vi "Action Name.vi"(11 "InitAction in":refnum<class "InitAction.lvclass">) -> (2 "Action Name":string)   [LabVIEW 2020, in "GPackTools.lvlib" / "InitAction.lvclass"]
uses:
  InitAction.lvclass
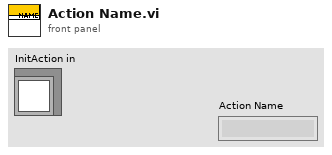
[diagram p1: front panel]
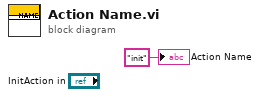
[diagram p0: block diagram]
diagram:
  "Action Name" <- "init" ("Action Name")
